vi "Line Detector Resample.vi"(6 "method":i32(ring)=1 items=["nearest", "linear", "spline", "cubic Hermite", "Lagrange"], 7 "Frequency":dbl[](array[numeric]), 8 "error in (no error)":errorcluster, 9 "Signal Y":dbl[](array[numeric]), 10 "Signal X":dbl[](array[numeric]), 11 "Line Detector Configuration":T1={"Peak width guess"=500.0, "Background removal"=enum."High-pass", "Smoothing"=enum."Low-pass", "Smooth window"=200.0, "Relative threshold"=0.2, "Finder algorithm"=enum."Wavelet", "Bgd window"=50000.0, "Spectrum recorder module name"="Spectrum Recorder", "Fit window"=1000.0, "Initial fit guess"=enum."Peak finder", "Follow\npeaks"=FALSE, "Re-sample"=nan} {"Re-sample" format="%#_6pHz"; "Fit window" format="%#_6pHz"; "Bgd window" format="%#_6pHz"; "Smooth window" format="%#_6pHz"; "Peak width guess" format="%#_6pHz"}) -> (0 "error out":errorcluster, 1 "Signal Y out":dbl[](array[numeric]), 2 "Signal X out":dbl[](array[numeric]), 5 "Frequency out":dbl[](array[numeric]))   [LabVIEW 2016]
uses:
  LabActor/Post-Processors/Line Detector/Resonance Detector Configuration.ctl
  <vilib>/gmath/NI_Gmath.lvlib
panel:
  # "Peak finder config"
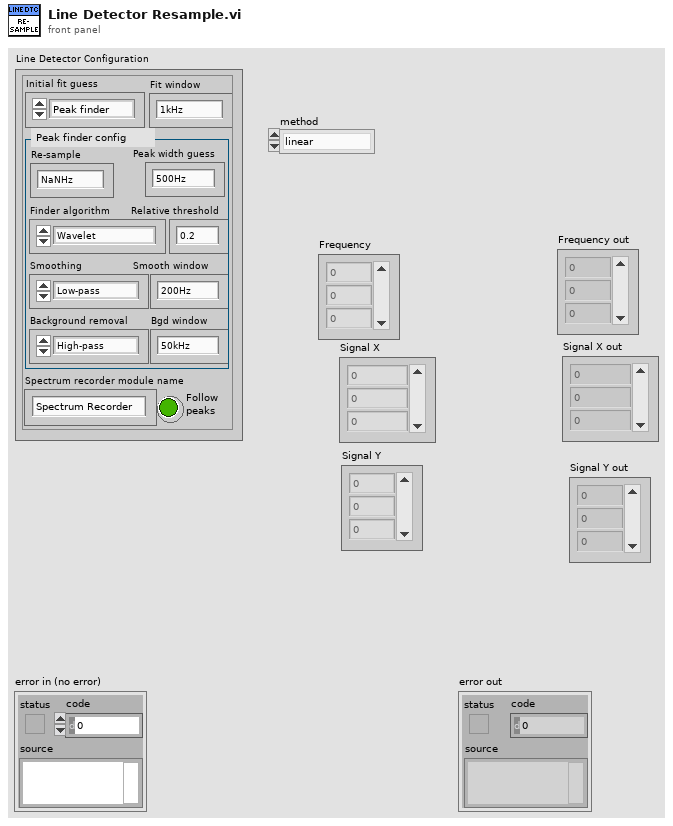
[diagram p1: front panel]
types:
  T1 = typedef "Resonance Detector Configuration.ctl" = cluster{"Peak width guess":dbl, "Background removal":enum16{"NONE", "High-pass", "Detrend"}, "Smoothing":enum16{"NONE", "Low-pass", "Denoise"}, "Smooth window":dbl, "Relative threshold":dbl, "Finder algorithm":enum16{"Basic", "Wavelet", "Wavelet+detrend"}, "Bgd window":dbl, "Spectrum recorder module name":string, "Fit window":dbl, "Initial fit guess":enum16{"Peak finder", "Last fit"}, "Follow\npeaks":bool, "Re-sample":dbl}
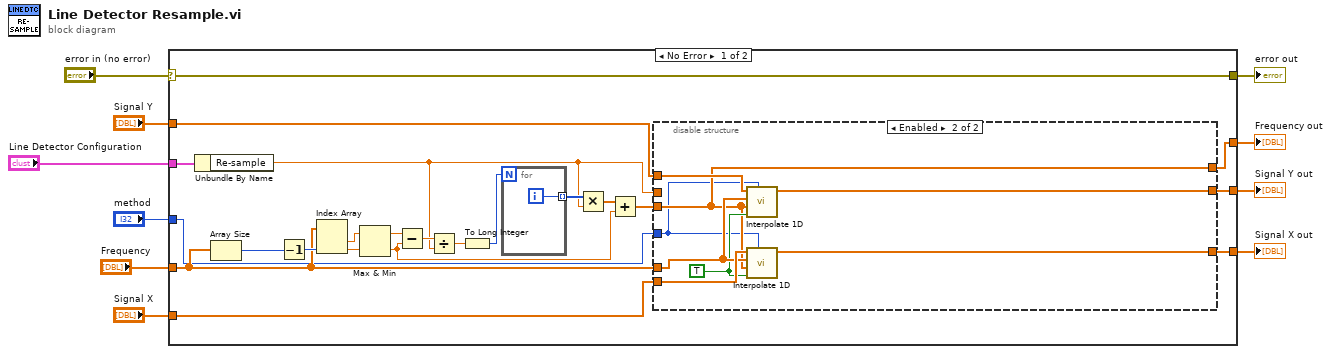
[diagram p0: block diagram]
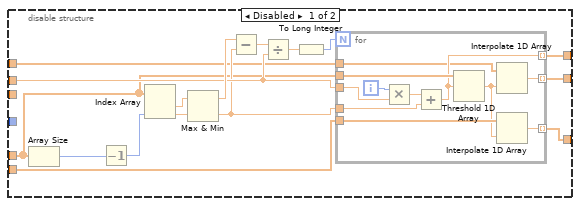
[diagram p2: hidden frame]
diagram:
  n1 = case shown="No Error" "error in (no error)" {
    selector: "error in (no error)" -> [w30 w72]
    tunnel: "Line Detector Configuration" -> [w32 _]
    tunnel: [w30 w72] -> w8
    tunnel: [w31 w71] -> w6
    tunnel: "Frequency" -> [w18 w71]
    tunnel: "Signal X" -> [w29 w70]
    tunnel: [w28 w70] -> w4
    tunnel: "Signal Y" -> [w27 w69]
    tunnel: [w26 w69] -> w2
    tunnel: "method" -> [w12 _]
    frame No Error {
      n2 = Unbundle By Name(w32) -> ("Re-sample"=w11:dbl)
      n3 = Array Size(array=w18) -> (size(s)=w19:i32)
      n4 = Decrement(x=w19) -> (x-1=w20:i32)
      n5 = Index Array(array=w18, index #2=w20) -> (element #1=w21:dbl, element #2=w22:dbl)  [unwired: 1 in]
      n6 = Max & Min(x=w21, y=w22) -> (max(x,y)=w23:dbl, min(x,y)=w15:dbl)
      n7 = Subtract(x=w23, y=w15) -> (x-y=w24:dbl)
      n8 = Divide(x=w24, y=w11) -> (x/y=w25:dbl)
      n9 = To Long Integer(number=w25) -> (32bit integer=w17:i32)
      n10 = for {
        N: w17 -> [_]
        tunnel: [w33] -> w14 mode=indexing
        i -> [w33]
      }
      n11 = Multiply(x=w14, y=w11) -> (x*y=w16:dbl[])
      n12 = Add(x=w16, y=w15) -> (x+y=w13:dbl[])
      n13 = disable-structure shown="Enabled" {
        disable-tunnel: w11 -> [w42 _]
        disable-tunnel: [w40 w64] -> w31
        disable-tunnel: w18 -> [w38 w66]
        disable-tunnel: w29 -> [w37 w68]
        disable-tunnel: [w36 w62] -> w28
        disable-tunnel: w27 -> [w35 w67]
        disable-tunnel: [w34 w63] -> w26
        disable-tunnel: w13 -> [_ w64]
        disable-tunnel: w12 -> [_ w61]
        frame Disabled {
          n14 = Array Size(array=w38) -> (size(s)=w49:i32)
          n15 = Decrement(x=w49) -> (x-1=w48:i32)
          n16 = Index Array(array=w38, index #2=w48) -> (element #1=w47:dbl, element #2=w46:dbl)  [unwired: 1 in]
          n17 = Max & Min(x=w47, y=w46) -> (max(x,y)=w45:dbl, min(x,y)=w41:dbl)
          n18 = Subtract(x=w45, y=w41) -> (x-y=w44:dbl)
          n19 = Divide(x=w44, y=w42) -> (x/y=w43:dbl)
          n20 = To Long Integer(number=w43) -> (32bit integer=w39:i32)
          n21 = for {
            N: w39 -> [_]
            tunnel: w42 -> [w60]
            tunnel: w41 -> [w58]
            tunnel: [w55] -> w40 mode=indexing
            tunnel: w38 -> [w56]
            tunnel: w37 -> [w54]
            tunnel: w35 -> [w53]
            tunnel: [w51] -> w36 mode=indexing
            tunnel: [w50] -> w34 mode=indexing
            i -> [w57]
            n22 = Multiply(x=w57, y=w60) -> (x*y=w59:dbl)
            n23 = Add(x=w59, y=w58) -> (x+y=w55:dbl)
            n24 = Threshold 1D Array(2:w55, 3:w56) -> (0:w52:dbl)  [unwired: 1 in]
            n25 = Interpolate 1D Array(1:w52, 2:w53) -> (0:w50:dbl)
            n26 = Interpolate 1D Array(1:w52, 2:w54) -> (0:w51:dbl)
          }
        }
        frame Enabled {
          w65 = TRUE ("X is monotonic")
          n27 = call <vilib>:"Interpolate 1D.vi"("method"=w61, "X is monotonic"=w65, "xi"=w64, "X"=w66, "Y"=w67) -> ("yi"=w63:dbl[])  [unwired: 4 in, 2 out]
          n28 = call <vilib>:"Interpolate 1D.vi"("method"=w61, "X is monotonic"=w65, "xi"=w64, "X"=w66, "Y"=w68) -> ("yi"=w62:dbl[])  [unwired: 4 in, 2 out]
        }
      }
    }
    frame Error {
    }
  }
  "error out" <- w8
  "Frequency out" <- w6
  "Signal X out" <- w4
  "Signal Y out" <- w2
